vi "Dark Sky Forecast Request.vi"(0 "API Key":string, 1 "Language":T9=enum."English", 5 "Latitude":dbl=42.3601 min=-90.0 max=90.0, 7 "Longitude":dbl=-71.0589 min=-180.0 max=180.0, 11 "error in":errorcluster, 12 "Units":T8="auto") -> (4 "Forecast Output":T1 {"Alerts"."alerts"."expires" format="%#_10g"; "Alerts"."alerts"."time" format="%#_10g"; "Daily Data"."daily"."data"."time" format="%#_10g"; "Hourly Data"."hourly"."data"."time" format="%#_10g"; "Minutely Data"."minutely"."data"."time" format="%#_10g"; "Current Data"."currently"."time" format="%#_10g"}, 15 "error out":errorcluster)   [LabVIEW 2017, in "Dark Sky Weather Data for LabVIEW.lvlib"]
doc: "Makes a Forecast request to the DarkSky API and interprets the result. A Forecast request returns the current weather conditions, a minute-by-minute forecast for the next hour (where available), an hour-by-hour forecast for the next 48 hours, and a day-by-day forecast for the next week - all for a given location in latitude and longitude coordinates.\n\nThis API call requires an API key (available free from DarkSky) and latitude + longitude coordinates. Use this alongside another API, for example from Google, to convert city names into coordinates if needed.\n\nMore info at https://darksky.net/dev/docs/forecast\n\nNeed an API Key? Visit: https://darksky.net/dev/ and sign up for free!"
uses:
  Dark Sky Weather Data for LabVIEW.lvlib
  Controls/Language Enum.ctl
  Controls/Units Enum.ctl
  Controls/Forecast Output.ctl
  Controls/Lat_Lon_TZ.ctl
  Controls/Forecast Current Data.ctl
  Controls/Forecast Minutely Data.ctl
  Controls/Forecast Hourly Data.ctl
  Controls/Forecast Daily Data.ctl
  Controls/Forecast Alert Data.ctl
  <vilib>/httpClient/LabVIEWHTTPClient.lvlib
panel:
  out "API Call URL":string
  # "Outputs - More Info at https://darksky.net/dev/docs/forecast"
  # "Inputs"
  # "Powered by Dark Sky"
  # "Need an API Key? Visit:\nhttps://darksky.net/dev/\nand sign up for free!"
  # "Instructions:\n-Enter an API Key\n-Enter Longitude, Latitude\n-Run the VI"
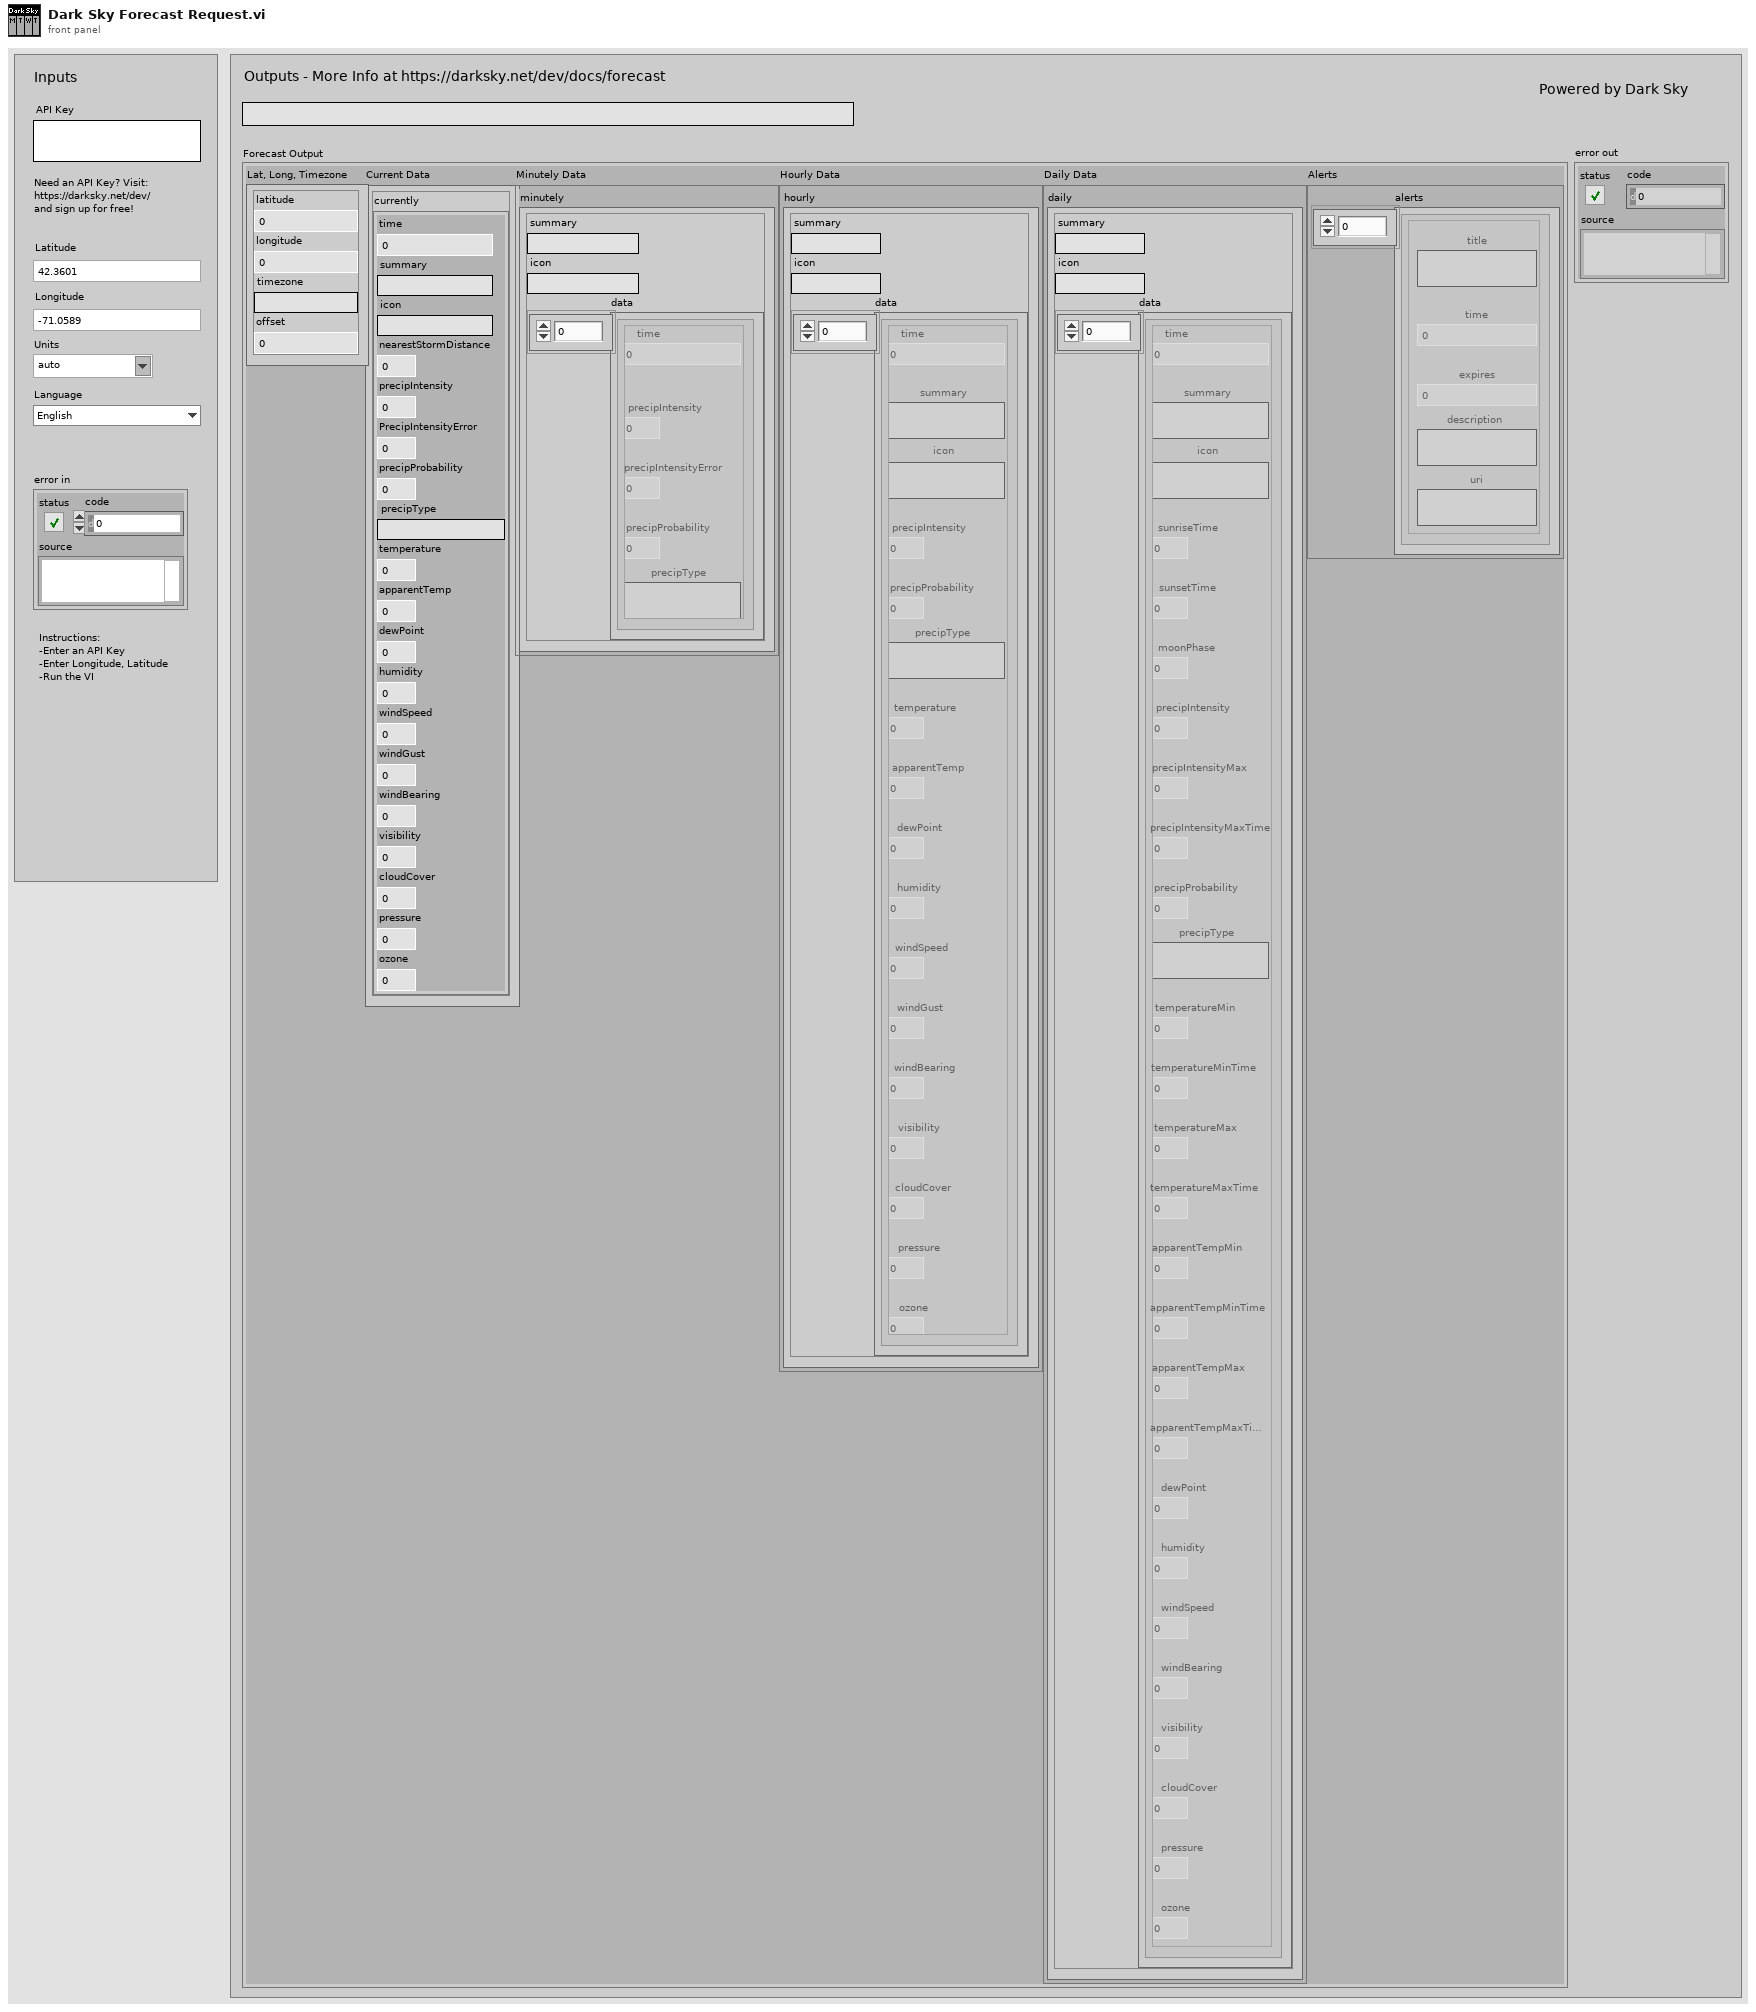
[diagram p1: front panel]
types:
  T1 = typedef "Dark Sky Weather Data for LabVIEW.lvlib/Forecast Output.ctl" = cluster{"Lat, Long, Timezone":T2, "Current Data":T3, "Minutely Data":T4, "Hourly Data":T5, "Daily Data":T6, "Alerts":T7}
  T2 = typedef "Dark Sky Weather Data for LabVIEW.lvlib/Lat_Lon_TZ.ctl" = cluster{"latitude":dbl, "longitude":dbl, "timezone":string, "offset":dbl}
  T3 = typedef "Dark Sky Weather Data for LabVIEW.lvlib/Forecast Current Data.ctl" = cluster{"currently":cluster{"time":dbl, "summary":string, "icon":string, "nearestStormDistance":dbl, "precipIntensity":dbl, "PrecipIntensityError":dbl, "precipProbability":dbl, "precipType":string, "temperature":dbl, "apparentTemp":dbl, "dewPoint":dbl, "humidity":dbl, "windSpeed":dbl, "windGust":dbl, "windBearing":dbl, "visibility":dbl, "cloudCover":dbl, "pressure":dbl, "ozone":dbl}}
  T4 = typedef "Dark Sky Weather Data for LabVIEW.lvlib/Forecast Minutely Data.ctl" = cluster{"minutely":cluster{"summary":string, "icon":string, "data":cluster{"time":dbl, "precipIntensity":dbl, "precipIntensityError":dbl, "precipProbability":dbl, "precipType":string}[]}}
  T5 = typedef "Dark Sky Weather Data for LabVIEW.lvlib/Forecast Hourly Data.ctl" = cluster{"hourly":cluster{"summary":string, "icon":string, "data":cluster{"time":dbl, "summary":string, "icon":string, "precipIntensity":dbl, "precipProbability":dbl, "precipType":string, "temperature":dbl, "apparentTemp":dbl, "dewPoint":dbl, "humidity":dbl, "windSpeed":dbl, "windGust":dbl, "windBearing":dbl, "visibility":dbl, "cloudCover":dbl, "pressure":dbl, "ozone":dbl}[]}}
  T6 = typedef "Dark Sky Weather Data for LabVIEW.lvlib/Forecast Daily Data.ctl" = cluster{"daily":cluster{"summary":string, "icon":string, "data":cluster{"time":dbl, "summary":string, "icon":string, "sunriseTime":dbl, "sunsetTime":dbl, "moonPhase":dbl, "precipIntensity":dbl, "precipIntensityMax":dbl, "precipIntensityMaxTime":dbl, "precipProbability":dbl, "precipType":string, "temperatureMin":dbl, "temperatureMinTime":dbl, "temperatureMax":dbl, "temperatureMaxTime":dbl, "apparentTempMin":dbl, "apparentTempMinTime":dbl, "apparentTempMax":dbl, "apparentTempMaxTime2":dbl, "dewPoint":dbl, "humidity":dbl, "windSpeed":dbl, "windBearing":dbl, "visibility":dbl, "cloudCover":dbl, "pressure":dbl, "ozone":dbl}[]}}
  T7 = typedef "Dark Sky Weather Data for LabVIEW.lvlib/Forecast Alert Data.ctl" = cluster{"alerts":cluster{"title":string, "time":dbl, "expires":dbl, "description":string, "uri":string}[]}
  T8 = typedef "Dark Sky Weather Data for LabVIEW.lvlib/Units Enum.ctl" = string
  T9 = typedef "Dark Sky Weather Data for LabVIEW.lvlib/Language Enum.ctl" = enum16{"Arabic", "Azerbaijani", "Belaursian", "Bulgarian", "Bosnian", "Catalan", "Czech", "German", "Greek", "English", "Spanish", "Estonian", "French", "Croatian", "Hungarian", "Indonesian", "Italian", "Icelandic", "Georgian", "Cornish", "Norwegian Bokmal", "Dutch", "Polish", "Portuguese", "Russian", "Slovak", "Slovenian", "Serbian", "Swedish", "Tetum", "Turkish", "Ukrainian", "simplified Chinese", "traditional Chinese"}
  T10 = typedef "LabVIEWHTTPClient.lvlib/ClientHandle.ctl" = refnum<k1>
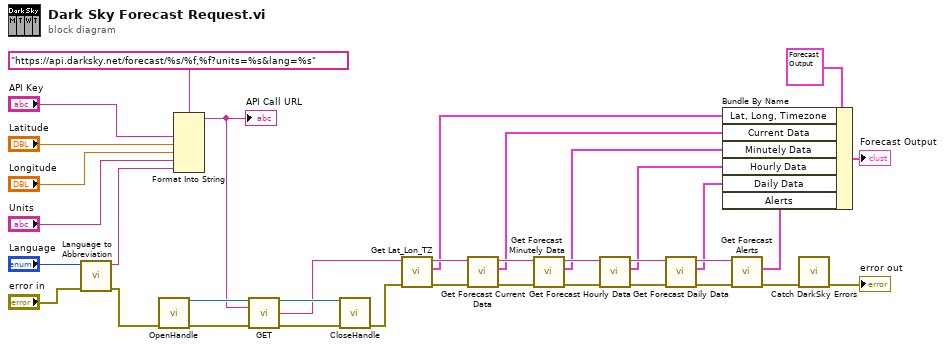
[diagram p0: block diagram]
diagram:
  n1 = call "Language to Abbreviation.vi"("error in (no error)"="error in", "Language"="Language") -> ("error out"=w34:errorcluster, "Language Abbreviation"=w28:string)  [unwired: 8 in]
  n2 = call <vilib>:"OpenHandle.vi"("error in (no error)"=w34) -> ("client handle out"=w25:T10, "error out"=w27:errorcluster)  [unwired: 13 in]
  n3 = Format Into String(format string="https://api.darksky.net/forecast/%s/%f,%f?units=%s&lang=%s", "API Key", "Latitude", "Longitude", "Units", w28) -> (resulting string=w23:string)  [unwired: 2 in, 1 out]
  "API Call URL" <- w23
  n4 = call <vilib>:"GET.vi"("client handle"=w25, "url"=w23, "error in (no error)"=w27) -> ("client handle out"=w24:T10, "body"=w22:string, "error out"=w26:errorcluster)  [unwired: 9 in, 1 out]
  n5 = call <vilib>:"CloseHandle.vi"("client handle"=w24, "error in (no error)"=w26) -> ("error out"=w21:errorcluster)  [unwired: 13 in]
  n6 = call "Get Lat_Lon_TZ.vi"("error in (no error)"=w21, "API Output"=w22) -> ("error out"=w20:errorcluster, "Lat, Long, Timezone"=w4:T2, "API Output (copy)"=w19:string)  [unwired: 7 in]
  n7 = call "Get Forecast Current Data.vi"("error in (no error)"=w20, "API Output"=w19) -> ("error out"=w18:errorcluster, "Current Data"=w5:T3, "API Output (copy)"=w17:string)  [unwired: 7 in]
  n8 = call "Get Forecast Minutely Data.vi"("error in (no error)"=w18, "API Output"=w17) -> ("error out"=w15:errorcluster, "Minutely Data"=w6:T4, "API Output (copy)"=w16:string)  [unwired: 7 in]
  n9 = call "Get Forecast Hourly Data.vi"("error in (no error)"=w15, "API Output"=w16) -> ("error out"=w13:errorcluster, "Hourly Data"=w7:T5, "API Output (copy)"=w14:string)  [unwired: 7 in]
  n10 = call "Get Forecast Daily Data.vi"("error in (no error)"=w13, "API Output"=w14) -> ("error out"=w12:errorcluster, "Daily Data"=w8:T6, "API Output (copy)"=w11:string)  [unwired: 7 in]
  n11 = call "Get Forecast Alerts.vi"("error in (no error)"=w12, "API Output"=w11) -> ("error out"=w2:errorcluster, "Alerts"=w9:T7)  [unwired: 7 in, 1 out]
  n12 = Bundle By Name(cluster=T1 {"Lat, Long, Timezone"={"latitude"=0.0, "longitude"=0.0, "timezone"="", "offset"=0.0}, "Current Data"={"currently"={"time"=0.0, "summary"="", "icon"="", "nearestStormDistance"=0.0, "precipIntensity"=0.0, "PrecipIntensityError"=0.0, "precipProbability"=0.0, "precipType"="", "temperature"=0.0, "apparentTemp"=0.0, "dewPoint"=0.0, "humidity"=0.0, "windSpeed"=0.0, "windGust"=0.0, "windBearing"=0.0, "visibility"=0.0, "cloudCover"=0.0, "pressure"=0.0, "ozone"=0.0}}, "Minutely Data"={"minutely"={"summary"="", "icon"="", "data"=[]}}, "Hourly Data"={"hourly"={"summary"="", "icon"="", "data"=[]}}, "Daily Data"={"daily"={"summary"="", "icon"="", "data"=[]}}, "Alerts"={"alerts"=[]}} ("Output Data"), "Lat, Long, Timezone"=w4, "Current Data"=w5, "Minutely Data"=w6, "Hourly Data"=w7, "Daily Data"=w8, "Alerts"=w9) -> (→"Forecast Output":T1)
  n13 = call "Catch DarkSky Errors.vi"("error in (no error)"=w2) -> ("error out"=→"error out":errorcluster)  [unwired: 10 in]
